vi "Test header flatten.vi"() -> ()   [LabVIEW 2021]
uses:
  typedef/FIFO Header.ctl
  <vilib>/CIF Foundation/CIF Utilities/DataTypes/Flatten U64.vi
  <vilib>/CIF Foundation/CIF Utilities/DataTypes/Flatten I64.vi
  <vilib>/CIF Foundation/CIF Utilities/DataTypes/Unflatten U64.vi
  <vilib>/CIF Foundation/CIF Utilities/DataTypes/Unflatten I64.vi
  <userlib>/_OpenG.lib/numeric/numeric.llb/Random Number Within Range - DBL__ogtk.vi
  ChannelCommon.lvlib
  <userlib>/_OpenG.lib/numeric/numeric.llb/openg_numeric__ogtk.lvlib
panel:
  out "Pass":bool
  out "Header out":T1
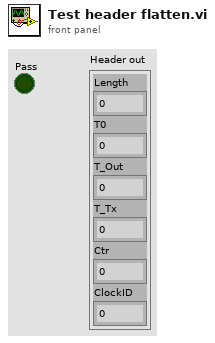
[diagram p1: front panel]
types:
  T1 = typedef "ChannelCommon.lvlib/FIFO Header.ctl" = cluster{"Length":u64, "T0":i64, "T_Out":i64, "T_Tx":i64, "Ctr":u64, "ClockID":u8}
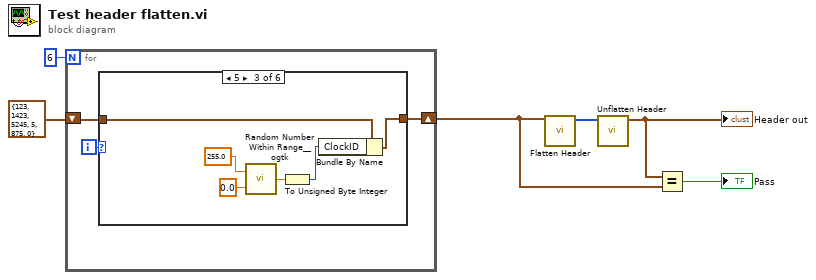
[diagram p0: block diagram]
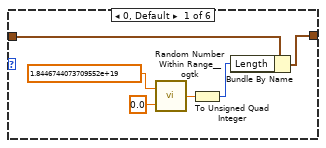
[diagram p2: hidden frame]
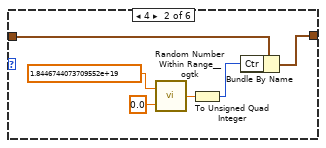
[diagram p3: hidden frame]
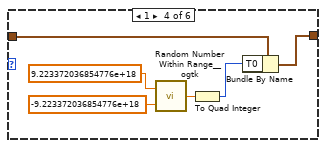
[diagram p4: hidden frame]
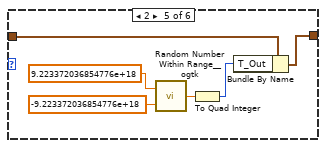
[diagram p5: hidden frame]
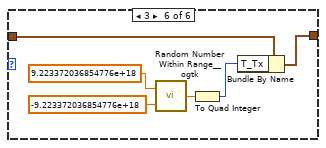
[diagram p6: hidden frame]
diagram:
  n1 = for {
    N: 6 -> [_]
    shift-right: [w7] -> w2
    shift-left: T1 {"Length"=123, "T0"=1423, "T_Out"=5245, "T_Tx"=5, "Ctr"=875, "ClockID"=0} ("Header in") -> [w8]
    i -> [w9]
    n2 = case shown="5" w9 {
      tunnel: w8 -> [w15 w21 w27 w33 w39 w45]
      tunnel: [w10 w16 w22 w28 w34 w40] -> w7
      frame 0, Default {
        n3 = call-poly <userlib>:"Random Number Within Range__ogtk.vi"("High"=1.8446744073709552e+19, "Low"=0.0) -> ("Random Number"=w12:dbl)  [unwired: 3 in]
        n4 = To Unsigned Quad Integer(1:w12) -> (0:w11:u64)
        n5 = Bundle By Name(cluster=w15, "Length"=w11) -> (w10:T1)
      }
      frame 4 {
        n6 = call-poly <userlib>:"Random Number Within Range__ogtk.vi"("High"=1.8446744073709552e+19, "Low"=0.0) -> ("Random Number"=w18:dbl)  [unwired: 3 in]
        n7 = To Unsigned Quad Integer(1:w18) -> (0:w17:u64)
        n8 = Bundle By Name(cluster=w21, "Ctr"=w17) -> (w16:T1)
      }
      frame 5 {
        n9 = call-poly <userlib>:"Random Number Within Range__ogtk.vi"("High"=255.0, "Low"=0.0) -> ("Random Number"=w24:dbl)  [unwired: 3 in]
        n10 = To Unsigned Byte Integer(number=w24) -> (unsigned 8bit integer=w23:u8)
        n11 = Bundle By Name(cluster=w27, "ClockID"=w23) -> (w22:T1)
      }
      frame 1 {
        n12 = call-poly <userlib>:"Random Number Within Range__ogtk.vi"("High"=9.223372036854776e+18, "Low"=-9.223372036854776e+18) -> ("Random Number"=w30:dbl)  [unwired: 3 in]
        n13 = To Quad Integer(1:w30) -> (0:w29:i64)
        n14 = Bundle By Name(cluster=w33, "T0"=w29) -> (w28:T1)
      }
      frame 2 {
        n15 = call-poly <userlib>:"Random Number Within Range__ogtk.vi"("High"=9.223372036854776e+18, "Low"=-9.223372036854776e+18) -> ("Random Number"=w36:dbl)  [unwired: 3 in]
        n16 = To Quad Integer(1:w36) -> (0:w35:i64)
        n17 = Bundle By Name(cluster=w39, "T_Out"=w35) -> (w34:T1)
      }
      frame 3 {
        n18 = call-poly <userlib>:"Random Number Within Range__ogtk.vi"("High"=9.223372036854776e+18, "Low"=-9.223372036854776e+18) -> ("Random Number"=w42:dbl)  [unwired: 3 in]
        n19 = To Quad Integer(1:w42) -> (0:w41:i64)
        n20 = Bundle By Name(cluster=w45, "T_Tx"=w41) -> (w40:T1)
      }
    }
  }
  n21 = call "Flatten Header.vi"("Header in"=w2) -> ("Flattened Data out"=w6:u8[])  [unwired: 10 in]
  n22 = call "Unflatten Header.vi"("Flattened Data in"=w6) -> ("Header out"=w3:T1)  [unwired: 9 in, 1 out]
  "Header out" <- w3
  n23 = Equal?(x=w3, y=w2) -> (x = y?=→"Pass":bool)
